vi "Robot Global Data.vi"() -> ()   [LabVIEW 2025]
doc: "This global VI can contain as many global variables as you need. To create a global variable, place a control on the panel, give it a good name. To read or write to it from a VI, drag the icon to the diagram of that VI. You can also drag from the project. Click on the node to change which global you access. You shouldn't have multiple locations writing to a global or it will cause a race-condition."
uses:
  <vilib>/Rock Robotics/WPI/Camera/WPI_CameraImageSize.ctl
  <vilib>/Rock Robotics/WPI/DriverStation/WPI_DriverStationRobotMode2.ctl
  Drive/Implementation/Drive Setpoints.ctl
  Drive/Implementation/Drive Operations.ctl
  swerve-template/Type Definitions/Data/Robot Velocities.ctl
  <vilib>/Rock Robotics/WPI/Framework/Command Status Info.ctl
  <vilib>/Rock Robotics/WPI/Framework/Completion Status.ctl
  <vilib>/Rock Robotics/WPI/Framework/Completion Notifier.ctl
  swerve-template/Type Definitions/Data/Pod Positions.ctl
  <vilib>/Rock Robotics/WPI/MotorControl/WPI_MotorControlDeviceRef.ctl
  <vilib>/Rock Robotics/WPI/MotorControl/WPI_MotorControlType.ctl
  <vilib>/Rock Robotics/SystemInterfaces/DIO/FPGA_DIOPWMChannel.ctl
  <vilib>/Rock Robotics/WPI/PWM/WPI_PWMDeadband.ctl
  <vilib>/Rock Robotics/SystemInterfaces/DIO/FPGA_DIOChannel.ctl
panel:
  in  "Limelight Name":string="/limelight-charged/"
  in  "Motor Data":T1[](array[typedef])
  in  "Pod Radius":dbl=1.0
  out "Pod Locations":T6 {"Right Back Position" format="%.2f"; "Right Front Position" format="%.2f"; "Left Back Position" format="%.2f"; "Left Front Position" format="%.2f"}
  out "Drive Controller Data":T13={"SubSystem Data"={"Operation"=enum."Reserve", "Robot Velocities"={"X Velocity"=0.0, "Y Velocity"=0.0, "Rotational \nVelocity"=0.0}, "Auto Data"={"Velocities"=[], "Positions"=[], [], "Zero Velocity?"=[], "dt array"=[]}}, {"Start Time (ms)"=1144712, "Iterations"=0}, {"Command Info"={"Name"="", "Status"=enum."Successful", "notifier out"=refnum}, "Description"="Default", "Default Command"={"Operation"=enum."Reserve", "Robot Velocities"={"X Velocity"=0.0, "Y Velocity"=0.0, "Rotational \nVelocity"=0.0}, "Auto Data"={"Velocities"=[], "Positions"=[], [], "Zero Velocity?"=[], "dt array"=[]}}, "queue out"=refnum, "Subsystem Name"="Drive"}}
  in  "Auto Done?":bool
  in  "Drive Conditions":cluster{"Field Centric":bool}={"Field Centric"=TRUE}
  in  "Robot Mode":T14
  in  "image size":T15=enum."320x240"
  in  "Enable Vision":bool
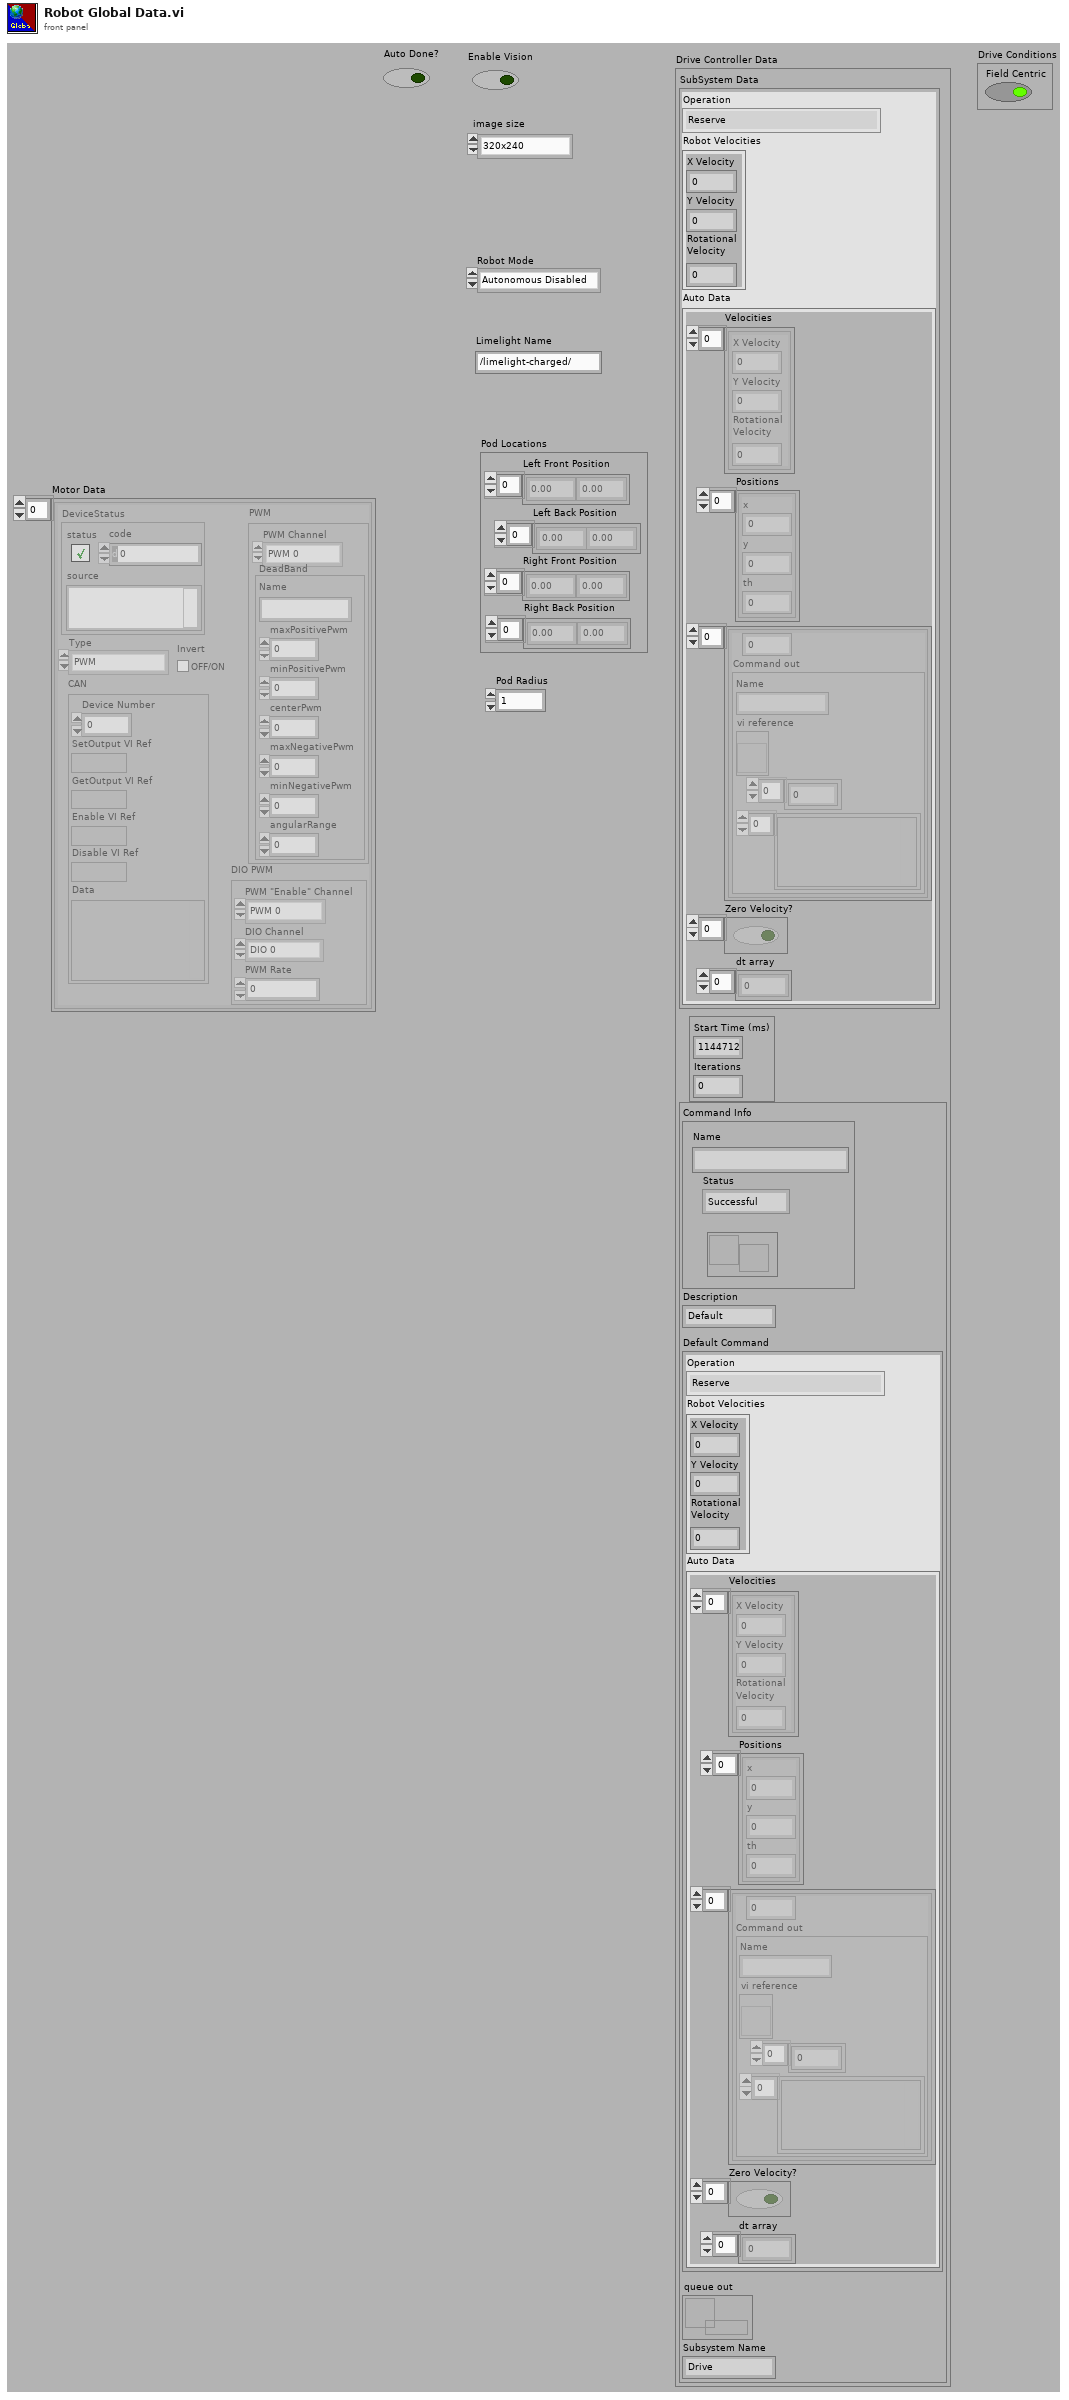
[diagram p1: front panel]
types:
  T1 = typedef "WPI_MotorControlDeviceRef.ctl" = cluster{"DeviceStatus":errorcluster, "Type":T2, "PWM":cluster{"PWM Channel":T3, "DeadBand":T4}, "CAN":cluster{"Device Number":u8, "SetOutput VI Ref":variant, "GetOutput VI Ref":variant, "Enable VI Ref":variant, "Disable VI Ref":variant, "Data":variant}, "Invert":bool, "DIO PWM":cluster{"PWM \"Enable\" Channel":T3, "DIOChannel":T5, "PWM Rate":dbl}}
  T2 = typedef "WPI_MotorControlType.ctl" = enum16{"PWM", "CAN", "DIO PWM"}
  T3 = typedef "FPGA_DIOPWMChannel.ctl" = enum8{"PWM 0", "PWM 1", "PWM 2", "PWM 3", "PWM 4", "PWM 5", "PWM 6", "PWM 7", "PWM 8", "PWM 9", "PWM MXP 0", "PWM MXP 1", "PWM MXP 2", "PWM MXP 3", "PWM MXP 4", "PWM MXP 5", "PWM MXP 6", "PWM MXP 7", "PWM MXP 8", "PWM MXP 9", "Invalid"}
  T4 = typedef "WPI_PWMDeadband.ctl" = cluster{"Name":string, "maxPositivePwm":i32, "minPositivePwm":i32, "centerPwm":i32, "maxNegativePwm":i32, "minNegativePwm":i32, "angularRange":u16}
  T5 = typedef "FPGA_DIOChannel.ctl" = enum8{"DIO 0", "DIO 1", "DIO 2", "DIO 3", "DIO 4", "DIO 5", "DIO 6", "DIO 7", "DIO 8", "DIO 9", "DIO MXP 0", "DIO MXP 1", "DIO MXP 2", "DIO MXP 3", "DIO MXP 4", "DIO MXP 5", "DIO MXP 6", "DIO MXP 7", "DIO MXP 8", "DIO MXP 9", "DIO MXP 10", "DIO MXP 11", "DIO MXP 12", "DIO MXP 13", "DIO MXP 14", "DIO MXP 15", "SPI Port CS1", "SPI Port CS2", "SPI Port CS3", "SPI Port MISO", "SPI Port MOSI", "Invalid"}
  T6 = typedef "Pod Positions.ctl" = cluster{"Left Front Position":dbl[], "Left Back Position":dbl[], "Right Front Position":dbl[], "Right Back Position":dbl[]}
  T7 = typedef "Drive Setpoints.ctl" = cluster{"Operation":T8, "Robot Velocities":T9, "Auto Data":cluster{"Velocities":T9[], "Positions":cluster{"x":dbl, "y":dbl, "th":dbl}[], cluster{dbl, "Command out":cluster{"Name":string, "vi reference":refnum<vi>, i32[], variant[]}}[], "Zero Velocity?":bool[], "dt array":dbl[]}}
  T8 = typedef "Drive Operations.ctl" = enum16{"Reserve", "Read Current", "Immediate", "Orbit", "Calibrate", "Auto"}
  T9 = typedef "Robot Velocities.ctl" = cluster{"X Velocity":dbl, "Y Velocity":dbl, "Rotational \nVelocity":dbl}
  T10 = typedef "Command Status Info.ctl" = cluster{"Name":string, "Status":T11, "notifier out":T12}
  T11 = typedef "Completion Status.ctl" = enum16{"Successful", "Aborted", "Incomplete"}
  T12 = typedef "Completion Notifier.ctl" = refnum<notifier>
  T13 = cluster{"SubSystem Data":T7, cluster{"Start Time (ms)":u32, "Iterations":i32}, cluster{"Command Info":T10, "Description":string, "Default Command":T7, "queue out":refnum<queue>, "Subsystem Name":string}}
  T14 = typedef "WPI_DriverStationRobotMode2.ctl" = enum16{"Autonomous Disabled", "Autonomous Enabled", "Teleop Disabled", "Teleop Enabled", "Disconnected", "Finish", "Test Disabled", "Test Enabled", "Emergency Stopped"}
  T15 = typedef "WPI_CameraImageSize.ctl" = enum16{"640x480", "320x240", "160x120", "Custom"}
diagram:
